vi "AVI-Initial and base file name.vi"(8 "error in (no error)":errorcluster, 11 "AVI file path & name":path) -> (0 "error out":errorcluster, 1 "Initial file name (increment = 1)":string, 2 "Base name is valid":bool, 3 "AVI file path":path, 4 "Base file name":string)   [LabVIEW 2017]
uses:
  Globals/gl_Time series viewer globals.vi
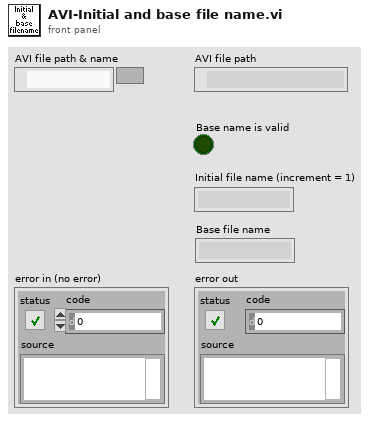
[diagram p1: front panel]
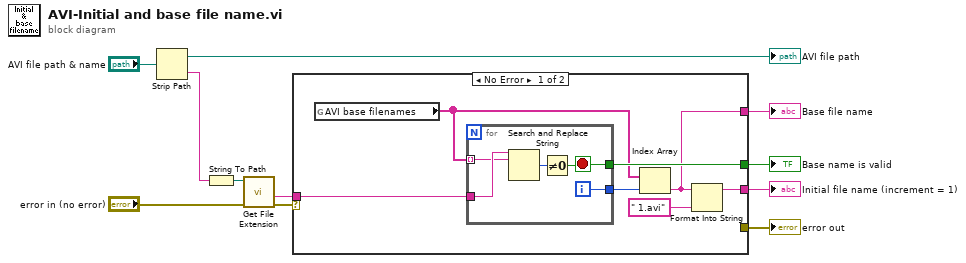
[diagram p0: block diagram]
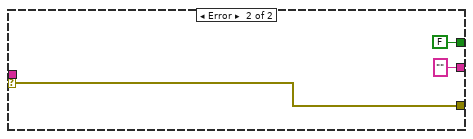
[diagram p2: hidden frame]
diagram:
  n1 = Strip Path(path="AVI file path & name") -> (stripped path=→"AVI file path":path, name=w9:string)
  n2 = String To Path(string=w9) -> (path=w6:path)
  n3 = call <vilib>:"Get File Extension.vi"("error in (no error)"="error in (no error)", "file"=w6) -> ("error out"=w3:errorcluster, "filename without extension"=w5:string)  [unwired: 5 in, 3 out]
  n4 = case shown="No Error" w3 {
    selector: w3 -> [_ w26]
    tunnel: [w17 ""] -> w11
    tunnel: w5 -> [w15 _]
    tunnel: [w14 FALSE] -> w4
    tunnel: [_ w26] -> w2
    tunnel: [w13 _] -> w1
    frame No Error {
      n5 = global read "gl_Time series viewer globals.vi" "AVI base filenames"() -> (w12:string[])
      n6 = for {
        tunnel: w12 -> [w22] mode=indexing
        tunnel: w15 -> [w23]
        tunnel: [w20] -> w18
        tunnel: [w19] -> w14
        i -> [w20]
        stop <- w19 stop-if-true
        n7 = Search and Replace String(input string=w23, search string=w22) -> (number of replacements=w21:i32)  [unwired: 6 in, 3 out]
        n8 = Not Equal To 0?(x=w21) -> (x != 0?=w19:bool)
      }
      n9 = Index Array(array=w12, index=w18) -> (element=w13:string)
      n10 = Format Into String(initial string=w13, " 1.avi" ("format string")) -> (resulting string=w17:string)  [unwired: 2 in, 1 out]
    }
    frame Error {
    }
  }
  "Initial file name (increment = 1)" <- w11
  "error out" <- w2
  "Base name is valid" <- w4
  "Base file name" <- w1
